vi "gui_dbg.vi"() -> ()   [LabVIEW 2019]
panel:
  in  "Settings Button":bool
  in  "Speed":i32(slide) scale=0.0..10.0
  in  "torque":i32(slide) scale=0.0..10.0
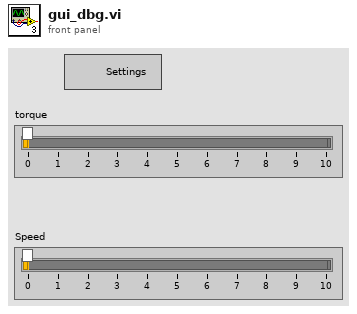
[diagram p1: front panel]
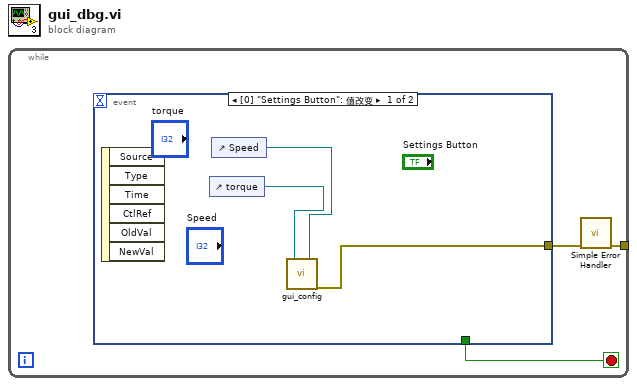
[diagram p0: block diagram]
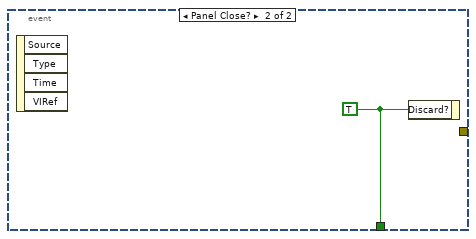
[diagram p2: hidden frame]
diagram:
  n1 = while {
    tunnel: [w1] -> _
    stop <- w3 stop-if-true
    n2 = event shown="[0] \"Settings Button\": 值改变" {
      selector: _ -> [_ _]
      dyn-events: _ -> [_ _]
      timeout: _ -> [_ _]
      tunnel: [_ w7] -> w3
      tunnel: [w4 _] -> w2
      event "Settings Button": Value Change {
        n3 = event-data() -> ()  [unwired: 1 in, 6 out]
        n4 = control-ref of="torque"() -> (w5:refnum<vi>)
        n5 = control-ref of="Speed"() -> (w6:refnum<vi>)
        n6 = call "gui_config.vi"("Torque"=w5, "Speed"=w6) -> ("error out"=w4:errorcluster)  [unwired: 10 in, 7 out]
      }
      event Panel Close? {
        w7 = TRUE ("Discard?")
        n7 = event-data() -> ()  [unwired: 1 in, 4 out]
        n8 = event-data("Discard?"=w7) -> ()  [unwired: 1 in, 1 out]
      }
    }
    n9 = call <vilib>:"Simple Error Handler.vi"("error in (no error)"=w2) -> ("error out"=w1:errorcluster)  [unwired: 4 in, 4 out]
  }
